vi "Initialize Chassis Tasks.vi"(8 "error in":errorcluster, 11 "Cfg wChassis":T1) -> (0 "error out":errorcluster, 3 "Chassis Tasks out":refnum<class "Chassis Tasks.lvclass">)   [LabVIEW 2012, in "Data Acquisition.lvlib" / "Chassis Tasks.lvclass"]
uses:
  Chassis Tasks.lvclass
  Custom Ctrls/Master Cfg/ge_Cfg wChassis.ctl
  Cfg Grandmaster/Class Chassis Cfg/ChassisCfg.lvclass
  Cfg Grandmaster/Class Chassis BOM/Chassis BOM.lvclass
  Common/Controls/TE_Designator.ctl
  Cfg Grandmaster/Class Chassis BOM/Chassis BOM.lvclass/Chassis BOM.ctl
  Class LS Only/LS Only.lvclass
  Class HS Only/HS Only.lvclass
  Class Master Slave/Master Slave.lvclass
  Chassis Tasks.lvclass/Chassis Tasks.ctl
  Cfg Grandmaster/Class Chassis BOM/Read Chassis Alias.vi
  Class DAQ Task/DAQ Task.lvclass
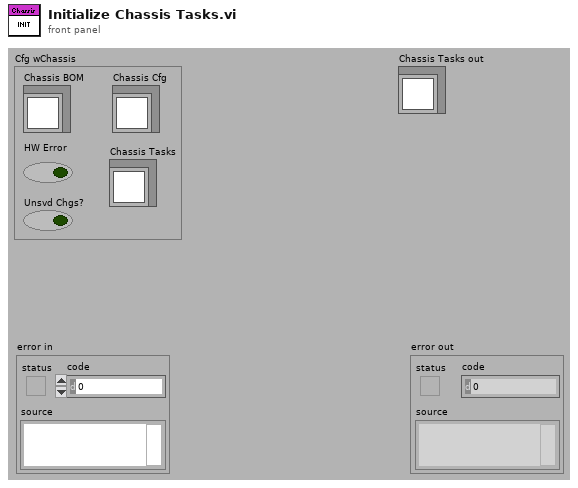
[diagram p1: front panel]
types:
  T1 = typedef "ge_Cfg wChassis.ctl" = cluster{"Chassis BOM":refnum<class "Chassis BOM.lvclass">, "Chassis Cfg":refnum<class "ChassisCfg.lvclass">, "Chassis Tasks":refnum<class "Chassis Tasks.lvclass">, "HW Error":bool, "Unsvd Chgs?":bool}
  T2 = typedef "TE_Designator.ctl" = enum16{"High Speed", "Low Speed"}
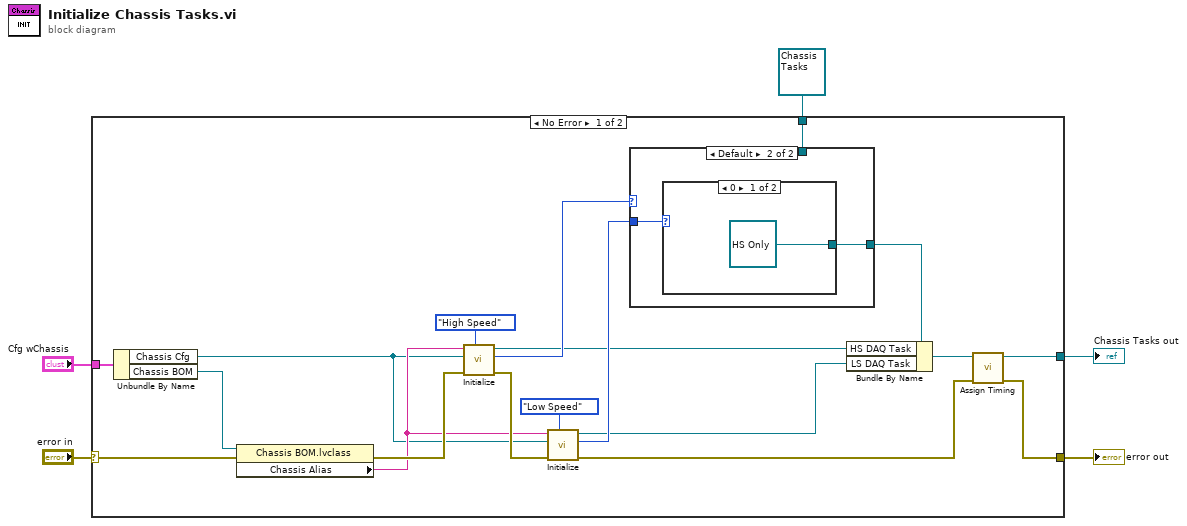
[diagram p0: block diagram]
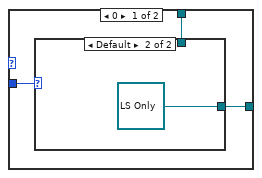
[diagram p2: hidden frame]
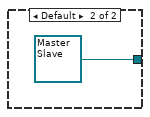
[diagram p4: hidden frame]
diagram:
  n1 = case shown="No Error" "error in" {
    selector: "error in" -> [w13 w35]
    tunnel: [w16 w35] -> w5
    tunnel: "Cfg wChassis" -> [w23 _]
    tunnel: [w15 w34] -> w2
    tunnel: refnum<class "Chassis Tasks.lvclass"> refnum ("Data Acquisition.lvlib:Chassis Tasks.lvclass") -> [w11 w34]
    frame No Error {
      n2 = Unbundle By Name(w23) -> ("Chassis Cfg"=w14:refnum<class "ChassisCfg.lvclass">, "Chassis BOM"=w12:refnum<class "Chassis BOM.lvclass">)
      n3 = property class="Chassis BOM.lvclass"(reference=w12, error in=w13) -> (error out=w24:errorcluster, "Chassis Alias"=w19:string)  [unwired: 1 out]
      n4 = call "Initialize.vi"("TimingEngine"=TE_Designator."High Speed", "error in (no error)"=w24, "Chassis Cfg"=w14, "Chassis Name"=w19) -> ("error out"=w20:errorcluster, "Num of Chans"=w18:i32, "DAQ Task out"=w7:refnum<class "DAQ Task.lvclass">)  [unwired: 5 in]
      n5 = call "Initialize.vi"("TimingEngine"=TE_Designator."Low Speed", "error in (no error)"=w20, "Chassis Cfg"=w14, "Chassis Name"=w19) -> ("error out"=w10:errorcluster, "Num of Chans"=w17:i32, "DAQ Task out"=w6:refnum<class "DAQ Task.lvclass">)  [unwired: 5 in]
      n6 = case shown="Default" w18 {
        tunnel: w17 -> [w27 w30]
        tunnel: [w26 w31] -> w9
        tunnel: w11 -> [w25 _]
        frame 0 {
          n7 = case shown="Default" w27 {
            tunnel: [w28 refnum<class "LS Only.lvclass"> refnum ("LS Only in")] -> w26
            tunnel: w25 -> [w28 _]
            frame 0 {
            }
            frame Default {
            }
          }
        }
        frame Default {
          n8 = case shown="0" w30 {
            tunnel: [refnum<class "HS Only.lvclass"> refnum ("HS Only in") refnum<class "Master Slave.lvclass"> refnum ("Master Slave in")] -> w31
            frame 0 {
            }
            frame Default {
            }
          }
        }
      }
      n9 = Bundle By Name(cluster=w9, "HS DAQ Task"=w7, "LS DAQ Task"=w6) -> (w8:refnum<class "Chassis Tasks.lvclass">)
      n10 = call-dynamic "Assign Timing.vi"("error in (no error)"=w10, "Chassis Tasks in"=w8) -> ("error out"=w16:errorcluster, "Chassis Tasks out"=w15:refnum<class "Chassis Tasks.lvclass">)  [unwired: 8 in]
    }
    frame Error {
    }
  }
  "error out" <- w5
  "Chassis Tasks out" <- w2
